vi "Renishaw-XL80_GetCancelPreHeat.vi"(8 "error in (no error)":errorcluster, 11 "Renishaw-XL80_EMU in":refnum<class "Renishaw-XL80_EMU.lvclass">) -> (0 "error out":errorcluster, 3 "Renishaw-XL80_EMU out":refnum<class "Renishaw-XL80_EMU.lvclass">)   [LabVIEW 2024, in "Renishaw-XL80_EMU.lvclass"]
uses:
  Renishaw-XL80_EMU.lvclass
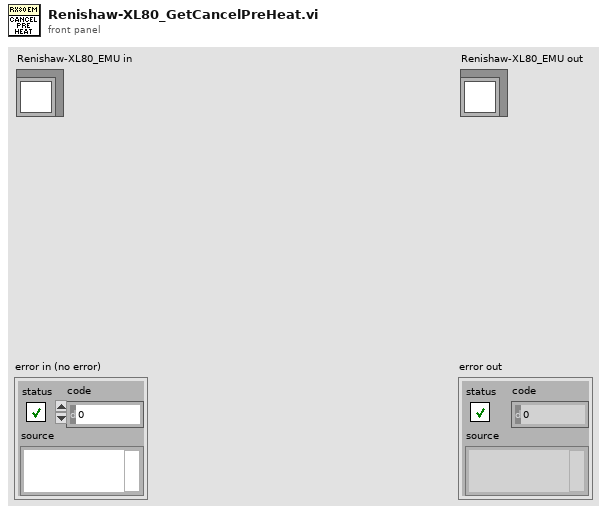
[diagram p1: front panel]
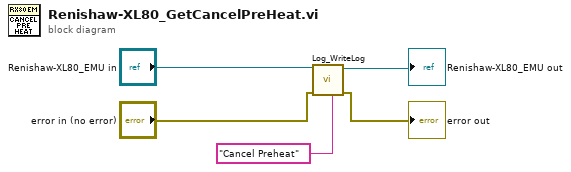
[diagram p0: block diagram]
diagram:
  n1 = call-dynamic "Log_WriteLog.vi"("Additional text"="Cancel Preheat", "error in (no error)"="error in (no error)", "Log in"="Renishaw-XL80_EMU in") -> ("error out"=→"error out":errorcluster, "Log out"=→"Renishaw-XL80_EMU out":refnum<class "Renishaw-XL80_EMU.lvclass">)  [unwired: 7 in]
